vi "set_xlim.vi"(6 "xlim":dbl[](array[numeric]), 8 "error in":errorcluster, 11 "figure (in)":refnum<vi>) -> (0 "error out":errorcluster, 3 "figure (out)":refnum<vi>)   [LabVIEW 2017]
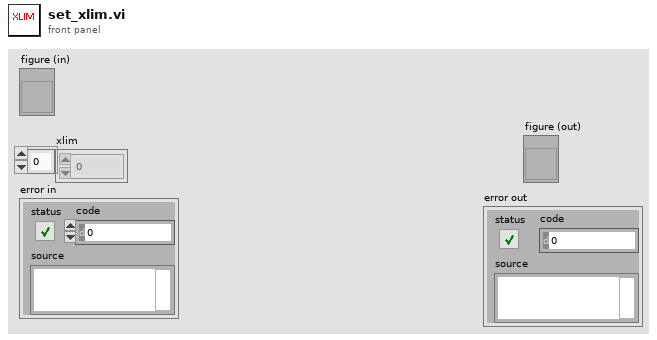
[diagram p1: front panel]
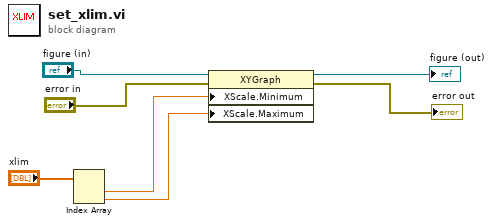
[diagram p0: block diagram]
diagram:
  n1 = Index Array(array="xlim") -> (element #1=w2:dbl, element #2=w1:dbl)  [unwired: 2 in]
  n2 = property on="Property Node" class="XYGraph"(reference="figure (in)", error in="error in", "XScale.Minimum"=w2, "XScale.Maximum"=w1) -> (reference out=→"figure (out)":refnum<vi>, error out=→"error out":errorcluster)
